vi "Examples Images 3.vi"() -> ()   [LabVIEW 2020, in "LcPictureBox.lvclass"]
uses:
  <userlib>/_LabVIEWCommon/LcPictureBox_class/LcPictureBox.lvclass
  <userlib>/_LabVIEWCommon/LcPictureBox_class/LcPictureBox.lvclass/LcPictureBox.ctl
  System.Windows.Forms
panel:
  out "Button":i32
  out "Y":i32
  out "X":i32
  out "ImageSize":cluster{"Width":i32, "Height":i32}
  out "Error Out":errorcluster
  in  "PictureBox":refnum<k24>(container)
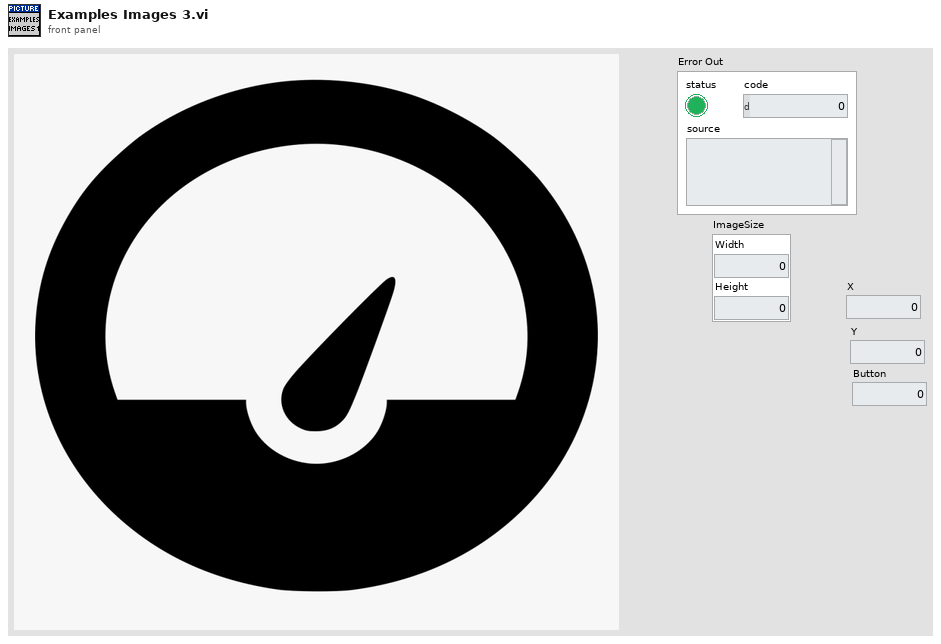
[diagram p1: front panel]
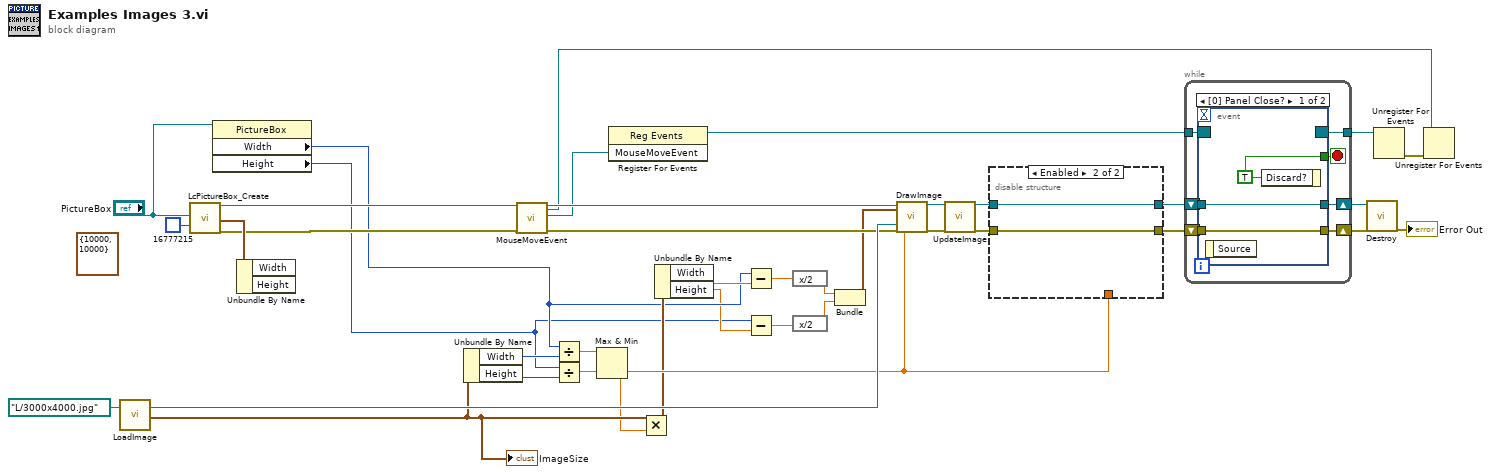
[diagram p0: block diagram]
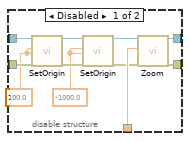
[diagram p2: hidden frame]
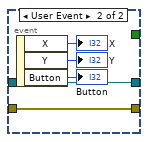
[diagram p3: hidden frame]
diagram:
  (unwired) cluster{"Width":i32, "Height":i32} {"Width"=10000, "Height"=10000} ("ImageSize(PictureBoxSize)")
  n1 = call <userlib>:"LoadImage.vi"("ImageFile"=path "L:/3000x4000.jpg") -> ("ImageOut"=w34:refnum<k24>, "ImageSize"=w12:cluster{"Width":i32, "Height":i32})  [unwired: 16 in, 1 out]
  "ImageSize" <- w12
  n2 = call <userlib>:"LcPictureBox_Create.vi"("PictureBox"="PictureBox", "BgColor(None)"=u32 16777215) -> ("reference out"=w23:refnum<class "LcPictureBox.lvclass">, "ImageSizeUsed"=w33:cluster{"Width":i32, "Height":i32}, "Error Out"=w22:errorcluster)  [unwired: 15 in]
  n3 = property on="Property Node" class="PictureBox"(reference="PictureBox") -> ("Width"=w8:i32, "Height"=w6:i32)  [unwired: 1 in, 2 out]
  n4 = Unbundle By Name(w33) -> ()  [unwired: 2 out]
  n5 = Unbundle By Name(w12) -> ("Width"=w32:i32, "Height"=w31:i32)
  n6 = call-dynamic "MouseMoveEvent.vi"("reference in"=w23, "error in (no error)"=w22) -> ("reference out"=w21:refnum<class "LcPictureBox.lvclass">, "Event Callback Refnum"=w15:refnum<k27>, "MouseMoveEvent"=w19:refnum<user-event>, "error out"=w20:errorcluster)  [unwired: 14 in]
  n7 = Divide(x=w8, y=w32) -> (x/y=w30:dbl)
  n8 = Divide(x=w6, y=w31) -> (x/y=w29:dbl)
  n9 = Max & Min(x=w30, y=w29) -> (min(x,y)=w11:dbl)  [unwired: 1 out]
  n10 = register-events(w19) -> (reference out=w18:refnum<event-registration>)  [unwired: 2 in, 1 out]
  n11 = Multiply(x=w12, y=w11) -> (x*y=w10:cluster{"Width":dbl, "Height":dbl})
  n12 = Unbundle By Name(w10) -> ("Width"=w9:dbl, "Height"=w7:dbl)
  n13 = Subtract(x=w8, y=w9) -> (x-y=w5:dbl)
  n14 = Subtract(x=w6, y=w7) -> (x-y=w4:dbl)
  n15 = expression code="x/2"(w5) -> (w3:dbl)
  n16 = expression code="x/2"(w4) -> (w2:dbl)
  n17 = Bundle(w3, w2) -> (w1:cluster{dbl, dbl})  [unwired: 1 in]
  n18 = call-dynamic "DrawImage.vi"("reference in"=w21, "UpperLeftCorner"=w1, "Image"=w34, "Error In"=w20, "ScaleFactor(1)"=w11) -> ("reference out"=w26:refnum<class "LcPictureBox.lvclass">, "Error Out"=w25:errorcluster)  [unwired: 13 in]
  n19 = call-dynamic "UpdateImage.vi"("reference in"=w26, "Error In"=w25) -> ("reference out"=w14:refnum<class "LcPictureBox.lvclass">, "Error Out"=w13:errorcluster)  [unwired: 14 in, 2 out]
  n20 = disable-structure shown="Enabled" {
    disable-tunnel: [w50 w52] -> w28
    disable-tunnel: [w49 w51] -> w27
    disable-tunnel: w11 -> [w48 _]
    disable-tunnel: w14 -> [w47 w52]
    disable-tunnel: w13 -> [w46 w51]
    frame Disabled {
      w42 = -1000.0 ("X")
      w43 = 100.0 ("X")
      n21 = call-dynamic "SetOrigin.vi"("reference in"=w47, "X"=w43, "Y"=w43, "Error In"=w46) -> ("reference out"=w45:refnum<class "LcPictureBox.lvclass">, "Error Out"=w44:errorcluster)  [unwired: 12 in, 2 out]
      n22 = call-dynamic "SetOrigin.vi"("reference in"=w45, "X"=w42, "Y"=w42, "Error In"=w44) -> ("reference out"=w41:refnum<class "LcPictureBox.lvclass">, "Error Out"=w40:errorcluster)  [unwired: 12 in, 2 out]
      n23 = call-dynamic "Zoom.vi"("reference in"=w41, "ZoomFactor"=w48, "Error In"=w40) -> ("reference out"=w50:refnum<class "LcPictureBox.lvclass">, "Error Out"=w49:errorcluster)  [unwired: 13 in, 2 out]
    }
    frame Enabled {
    }
  }
  n24 = while {
    shift-right: [w58] -> w36
    shift-left: w28 -> [w57]
    shift-right: [w59] -> w37
    shift-left: w27 -> [w56]
    tunnel: w18 -> [w55]
    tunnel: [w54] -> w17
    stop <- w53 stop-if-true
    n25 = event shown="[0] Panel Close?" {
      selector: w55 -> [_ _]
      dyn-events: [_ _] -> w54
      timeout: _ -> [_ _]
      tunnel: w56 -> [w62 w63]
      tunnel: [w62 w63] -> w59
      tunnel: w57 -> [w61 w64]
      tunnel: [w61 w64] -> w58
      tunnel: [w60 _] -> w53
      event Panel Close? {
        w60 = TRUE ("Discard?")
        n26 = event-data() -> ()  [unwired: 1 in, 1 out]
        n27 = event-data("Discard?"=w60) -> ()  [unwired: 1 in, 1 out]
      }
      event User Event {
        n28 = event-data() -> ("X"=→"X":i32, "Y"=→"Y":i32, "Button"=→"Button":i32)  [unwired: 1 in]
      }
    }
  }
  n29 = call-dynamic "Destroy.vi"("reference in"=w36, "Error In"=w37) -> ("Error Out"=→"Error Out":errorcluster)  [unwired: 16 in, 1 out]
  n30 = Unregister For Events(event registration refnum=w17) -> (error out=w16:errorcluster)  [unwired: 1 in]
  n31 = Unregister For Events(event registration refnum=w15, error in=w16) -> ()  [unwired: 1 out]
